vi "PixmapCtrlDefault.vi"(1 "image data":T1) -> (0 "Pause if TRUE":bool)   [LabVIEW 2017]
doc: "Displays the pixmap."
uses:
  <vilib>/picture/picture.llb/imagedata.ctl
panel:
  out "Bad picture":T2
  out "picture out":picture
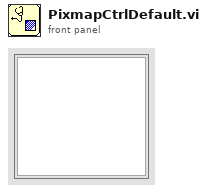
[diagram p1: front panel]
types:
  T1 = typedef "imagedata.ctl" = cluster{"image type":i32, "image depth":i32, "image":u8[], "mask":u8[], "colors":u32[], "Rectangle":cluster{"left":i16, "top":i16, "right":i16, "bottom":i16}}
  T2 = cluster{"Picture is empty or invalid":string, "Left:":i16, "Top:":i16, "Right:":i16, "Bottom:":i16}
  T3 = enum16{"Always On", "Always Off", "Off While Running"}
  T4 = typedef "LVBoundsTypeDef.ctl" = cluster{"Width":u32, "Height":u32}
  T5 = cluster{string, "left":i16, "top":i16, "right":i16, "bottom":i16}
  T6 = typedef "LVRectTypeDef.ctl" = cluster{"Left":i16, "Top":i16, "Right":i16, "Bottom":i16}
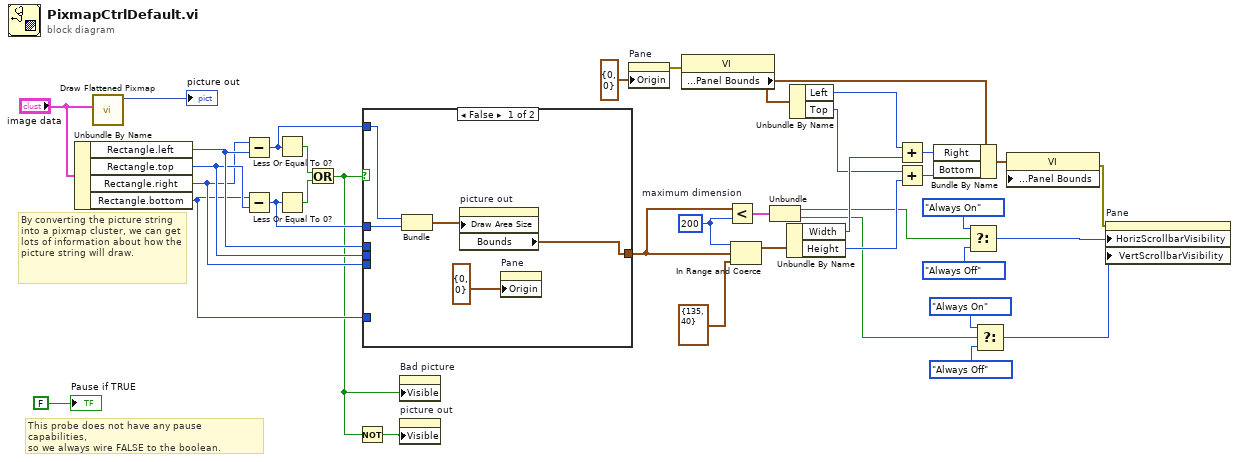
[diagram p0: block diagram]
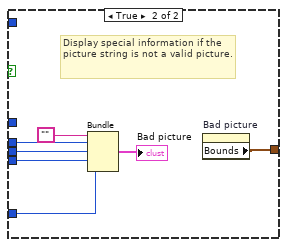
[diagram p2: hidden frame]
diagram:
  w17 = i16 200  # maximum dimension
  # "This probe does not have any pause capabilities,\nso we always wire FALSE to the boolean."
  # "By converting the picture string into a pixmap cluster, we can get lots of information about how the picture string will draw."
  n1 = Unbundle By Name("image data") -> ("Rectangle.left"=w34:i16, "Rectangle.top"=w33:i16, "Rectangle.right"=w32:i16, "Rectangle.bottom"=w31:i16)
  n2 = call <vilib>:"Draw Flattened Pixmap.vi"("image data"="image data") -> ("new picture"=→"picture out":picture)  [unwired: 8 in]
  n3 = Subtract(x=w32, y=w34) -> (x-y=w30:i16)
  n4 = Subtract(x=w31, y=w33) -> (x-y=w29:i16)
  n5 = Less Or Equal To 0?(x=w30) -> (x <= 0?=w36:bool)
  n6 = Less Or Equal To 0?(x=w29) -> (x <= 0?=w35:bool)
  n7 = Or(x=w36, y=w35) -> (x .or. y?=w19:bool)
  n8 = Not(x=w19) -> (.not. x?=w18:bool)
  n9 = case shown="False" w19 {
    tunnel: w34 -> [_ w48]
    tunnel: w33 -> [_ w47]
    tunnel: w32 -> [_ w46]
    tunnel: w31 -> [_ w45]
    tunnel: [w39 w43] -> w16
    tunnel: w30 -> [w40 _]
    tunnel: w29 -> [w41 _]
    frame False {
      n10 = Bundle(w40, w41) -> (w42:cluster{i16, i16})  [unwired: 1 in]
      n11 = property on="picture out" class="Pict"("Draw Area Size"=w42) -> ("Bounds"=w39:T4)  [unwired: 2 in, 2 out]
      n12 = property on="Pane" class="Pane"("Origin"=cluster{"Horizontal":i16, "Vertical":i16} {"Horizontal"=0, "Vertical"=0}) -> ()  [unwired: 2 in, 2 out]
    }
    frame True {
      # "Display special information if the picture string is not a valid picture."
      n13 = Bundle("", "left"=w48, "top"=w47, "right"=w46, "bottom"=w45) -> (→"Bad picture":T5)  [unwired: 1 in]
      n14 = property on="Bad picture" class="Clust (strict)"() -> ("Bounds"=w43:T4)  [unwired: 2 in, 2 out]
    }
  }
  n15 = property on="Bad picture" class="Clust (strict)"("Visible"=w19) -> ()  [unwired: 2 in, 2 out]
  n16 = property on="picture out" class="Pict"("Visible"=w18) -> ()  [unwired: 2 in, 2 out]
  n17 = property on="Pane" class="Pane"("Origin"=cluster{"Horizontal":i16, "Vertical":i16} {"Horizontal"=0, "Vertical"=0} ("Front Panel Window:Origin")) -> (error out=w7:errorcluster)  [unwired: 2 in, 1 out]
  n18 = property class="VI"(error in=w7) -> ("Front Panel Window:Panel Bounds"=w24:T6)  [unwired: 1 in, 2 out]
  n19 = Less?(x=w16, y=w17) -> (x < y?=w15:cluster{"Width":bool, "Height":bool})
  n20 = In Range and Coerce(upper limit=w17, x=w16, lower limit=cluster{"Width":u32, "Height":u32} {"Width"=135, "Height"=40}) -> (coerced(x)=w20:T4)  [unwired: 1 out]
  n21 = Unbundle(w15) -> ("Width"=w2:bool, "Height"=w1:bool)
  n22 = Unbundle By Name(w20) -> ("Width"=w27:u32, "Height"=w25:u32)
  n23 = Unbundle By Name(w24) -> ("Left"=w28:i16, "Top"=w26:i16)
  n24 = Add(x=w28, y=w27) -> (x+y=w23:u32)
  n25 = Add(x=w26, y=w25) -> (x+y=w22:u32)
  n26 = Bundle By Name(cluster=w24, "Right"=w23, "Bottom"=w22) -> (w21:T6)
  n27 = Select(t=T3."Always On" ("Horizontal Scrollbar Visibility"), s=w2, f=T3."Always Off" ("Horizontal Scrollbar Visibility")) -> (s? t:f=w8:T3)
  n28 = Select(t=T3."Always On" ("Horizontal Scrollbar Visibility"), s=w1, f=T3."Always Off" ("Horizontal Scrollbar Visibility")) -> (s? t:f=w3:T3)
  n29 = property class="VI"("Front Panel Window:Panel Bounds"=w21) -> (error out=w11:errorcluster)  [unwired: 2 in, 1 out]
  n30 = property on="Pane" class="Pane"(error in=w11, "HorizScrollbarVisibility"=w8, "VertScrollbarVisibility"=w3) -> ()  [unwired: 1 in, 2 out]
  "Pause if TRUE" <- FALSE ("Boolean")
